vi "sawtooth-wave-gen.vi"(8 "floor":dbl, 9 "limit":dbl=100.0, 10 "i":dbl=1.0, 11 "current-val":dbl) -> (3 "output":dbl)   [LabVIEW 2024]
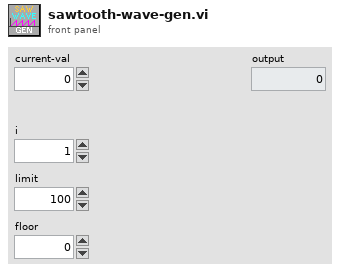
[diagram p1: front panel]
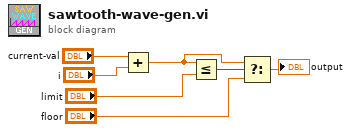
[diagram p0: block diagram]
diagram:
  n1 = Add(x="current-val", y="i") -> (x+y=w6:dbl)
  n2 = Less Or Equal?(x=w6, y="limit") -> (x <= y?=w5:bool)
  n3 = Select(t=w6, s=w5, f="floor") -> (s? t:f=→"output":dbl)
